vi "GetSetHighLimit.vi"(0 "VISA resource name":refnum<visa-resource-name>, 5 "get/set":T2, 7 "Channel Number (1-4)":T1=1 items=["Channel 1"=1, "Channel 2"=2, "Channel 3"=3, "Channel 4"=4], 9 "Setpoint":dbl min=-200.0 max=300.0 step=1.0 format="%.1f", 11 "error in":errorcluster) -> (4 "VISA resource name out":refnum<visa-resource-name>, 6 "Setpoint string":string, 8 "Setpoint":dbl format="%.1f", 15 "error out":errorcluster)   [LabVIEW 2023, in "Thermotron 8800.lvlib"]
doc: "PALH\nCommand name: Send high process alarm limit\nCommand type: Program status\nDescription: Queries the 8800 for a channel’s high process alarm limit. The 8800 sends an integer\nindicating the alarm limit.\nSyntax: PALHn?\nWhere n is a channel number.\nData type: Integer\nQuery example: PALH1?\n8800 response: 100 (The channel 1 high process alarm limit is 100.)"
uses:
  Thermotron 8800.lvlib
  Private/get set.ctl
  Private/AnalogInputChannelNumber 1-4.ctl
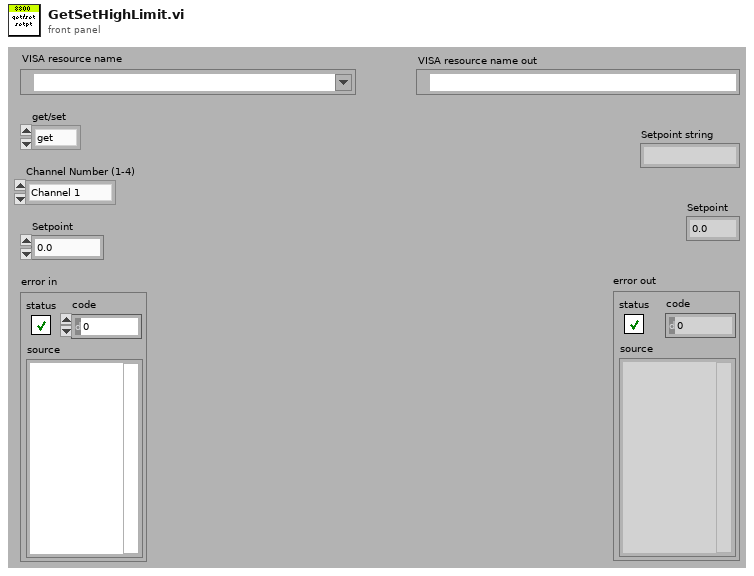
[diagram p1: front panel]
types:
  T1 = typedef "Thermotron 8800.lvlib/AnalogInputChannelNumber 1-4.ctl" = u16
  T2 = typedef "Thermotron 8800.lvlib/get set.ctl" = enum16{"get", "set"}
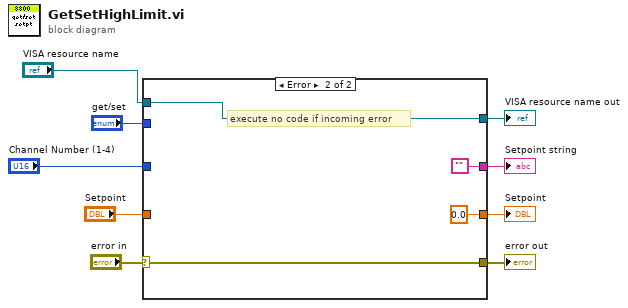
[diagram p0: block diagram]
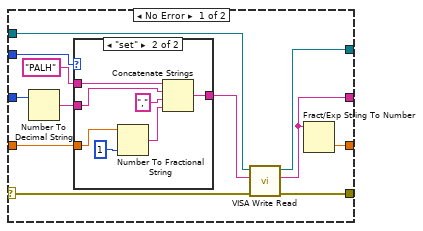
[diagram p2: hidden frame]
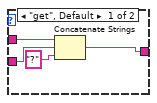
[diagram p3: hidden frame]
diagram:
  n1 = case shown="Error" "error in" {
    selector: "error in" -> [w11 w35]
    tunnel: "get/set" -> [w21 _]
    tunnel: [w12 ""] -> w3
    tunnel: [w10 w35] -> w6
    tunnel: [w13 w36] -> w8
    tunnel: "VISA resource name" -> [w15 w36]
    tunnel: "Setpoint" -> [w19 _]
    tunnel: [w18 0.0] -> w2
    tunnel: "Channel Number (1-4)" -> [w17 _]
    frame No Error {
      n2 = Number To Decimal String(number=w17) -> (decimal integer string=w16:string)  [unwired: 1 in]
      n3 = case shown="\"set\"" w21 {
        tunnel: "PALH" ("8800 Command") -> [w24 w32]
        tunnel: [w25 w31] -> w14
        tunnel: w19 -> [_ w30]
        tunnel: w16 -> [w22 w26]
        frame "get", Default {
          n4 = Concatenate Strings(w24, w22, "?" ("8800 Command")) -> (w25:string)
        }
        frame "set" {
          n5 = Number To Fractional String(number=w30, precision (6)=i16 1) -> (F-format string=w28:string)  [unwired: 2 in]
          n6 = Concatenate Strings(w32, w26, "," ("string"), w28) -> (w31:string)
        }
      }
      n7 = call "VISA Write Read.vi"("error in (no error)"=w11, "8800 Command"=w14, "VISA Refnum in"=w15) -> ("error out"=w10:errorcluster, "read buffer"=w12:string, "VISA Refnum out"=w13:refnum<visa-resource-name>)  [unwired: 6 in]
      n8 = Fract/Exp String To Number(string=w12) -> (number=w18:dbl)  [unwired: 3 in, 1 out]
    }
    frame Error {
      # "execute no code if incoming error"
    }
  }
  "VISA resource name out" <- w8
  "error out" <- w6
  "Setpoint string" <- w3
  "Setpoint" <- w2
